vi "Do.vi"(8 "error in (no error)":errorcluster, 10 "Actor in":refnum<class "Actor.lvclass">, 11 "Connected Msg":refnum<class "Connected Msg.lvclass">) -> (0 "error out":errorcluster, 2 "Actor out":refnum<class "Actor.lvclass">)   [LabVIEW 2021, in "Client.lvlib" / "Connected Msg.lvclass"]
doc: "This VI delivers the message to the actor by calling the appropriate method(s) on the actor."
uses:
  Connected Msg.lvclass
  C:/Program Files/National Instruments/LabVIEW 2021/vi.lib/NI/Actors/Network Endpoint Actors/Nested Endpoint/Nested Endpoint Messages/Connected Msg/Connected Msg.lvclass
  <vilib>/ActorFramework/Actor/Actor.lvclass
  Client/Client.lvclass
  C:/Program Files/National Instruments/LabVIEW 2021/vi.lib/ActorFramework/Actor/Actor.lvclass
  <vilib>/NI/Actors/Network Endpoint Actors/Nested Endpoint/Nested Endpoint Messages/Connected Msg/Connected Msg.lvclass/Connected Msg.ctl
  34700b1e-4b1b-4205-ab4b-28631ba2a4c6.vi
  <vilib>/NI/Actors/Network Endpoint Actors/Nested Endpoint/Nested Endpoint Messages/Connected Msg/Connected Msg.lvclass
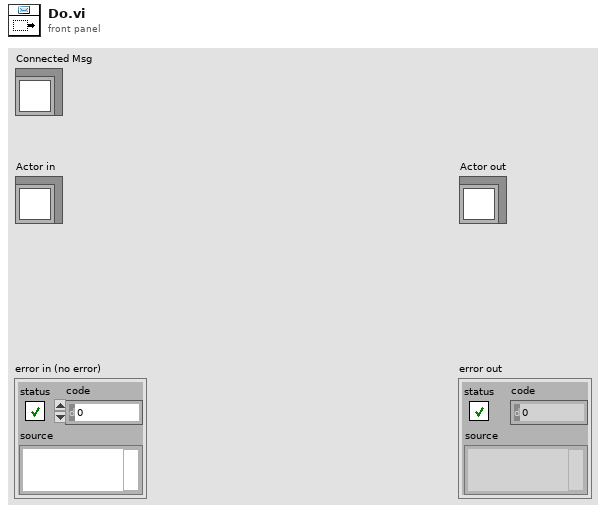
[diagram p1: front panel]
types:
  T1 = cluster{"Endpoint Enqueuer":refnum<class "Message Enqueuer.lvclass">, "Message Stream":refnum<class "Message Stream.lvclass">}
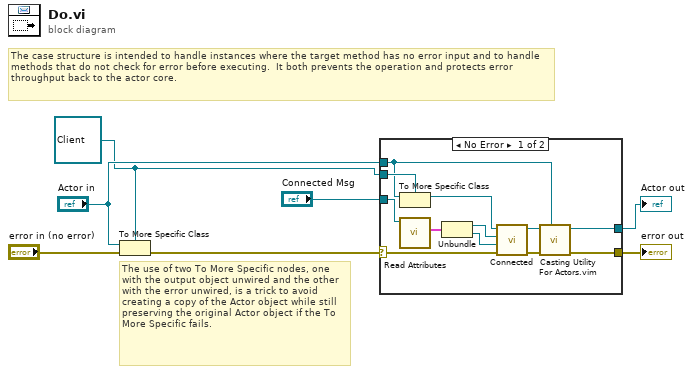
[diagram p0: block diagram]
diagram:
  w2 = refnum<class "Client.lvclass"> refnum ("Actor in")
  # "The use of two To More Specific nodes, one with the output object unwired and the other with the error unwired, is a trick to avoid creating a copy of the Actor object while still preserving the original Actor object if the To More Specific fails."
  # "The case structure is intended to handle instances where the target method has no error input and to handle methods that do not check for error before executing.  It both prevents the operation and protects error throughput back to the actor core."
  n1 = To More Specific Class(target class=w2, reference="Actor in", error in="error in (no error)") -> (error out=w6:errorcluster)  [unwired: 1 out]
  n2 = case shown="No Error" w6 {
    selector: w6 -> [w19 w21]
    tunnel: [w11 w21] -> w5
    tunnel: [w10 w20] -> w4
    tunnel: "Actor in" -> [w14 w20]
    tunnel: w2 -> [w15 _]
    tunnel: "Connected Msg" -> [w16 _]
    frame No Error {
      n3 = To More Specific Class(target class=w15, reference=w14) -> (specific class reference=w18:refnum<class "Client.lvclass">)  [unwired: 1 in, 1 out]
      n4 = call <vilib>:"Read Attributes.vi"("Connected Msg"=w16) -> ("Payload"=w17:T1)  [unwired: 10 in]
      n5 = Unbundle(w17) -> ("Endpoint Enqueuer"=w9:refnum<class "Message Enqueuer.lvclass">, "Message Stream"=w8:refnum<class "Message Stream.lvclass">)
      n6 = call "Connected.vi"("error in (no error)"=w19, "Message Stream"=w8, "Endpoint Enqueuer"=w9, "Client in"=w18) -> ("error out"=w12:errorcluster, "Client out"=w13:refnum<class "Client.lvclass">)  [unwired: 6 in]
      n7 = call "Casting Utility For Actors.vim"("type"=w14, "error in (no error)"=w12, "Actor in"=w13) -> ("error out"=w11:errorcluster, "Actor out"=w10:refnum<class "Actor.lvclass">)  [unwired: 7 in]
    }
    frame Error {
      # "If type check fails, pass the original object out again."
    }
  }
  "error out" <- w5
  "Actor out" <- w4
